vi "Edit Master Gas Mixture.vi"(8 "error in":errorcluster, 11 "Gas Info":T1) -> (0 "error out":errorcluster, 2 "Cancel?":bool, 3 "Gas Info Out":T1)   [LabVIEW 2015]
uses:
  Tests/Controls/Gas Info.ctl
panel:
  in  "Time (s)":u32
  in  "Cancel Button":bool
  in  "OK Button":bool
  in  "PPM":dbl
  in  "Gas":string(combo)
  # "Gas Configuration"
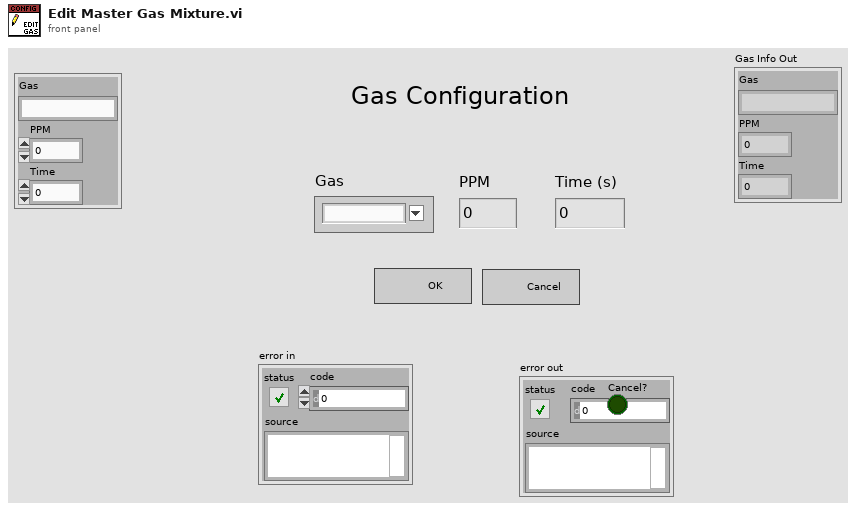
[diagram p1: front panel]
types:
  T1 = typedef "Gas Info.ctl" = cluster{"Gas":string, "PPM":dbl, "Time":u32}
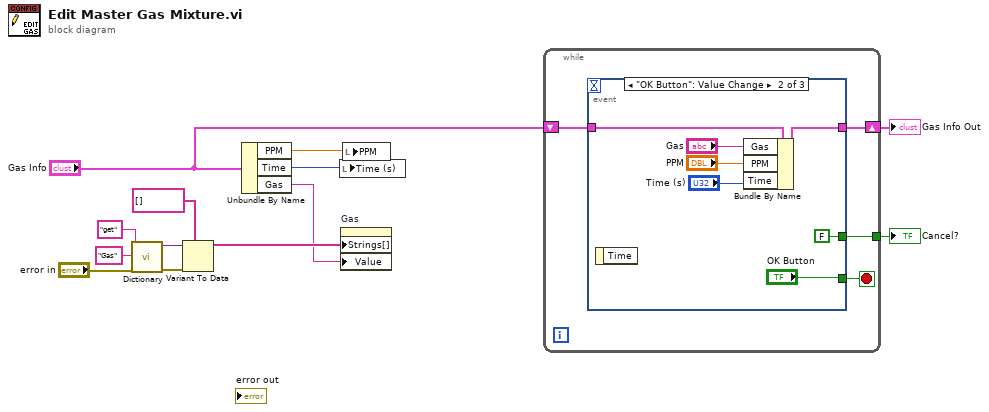
[diagram p0: block diagram]
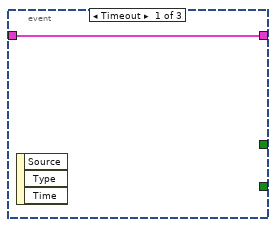
[diagram p2: hidden frame]
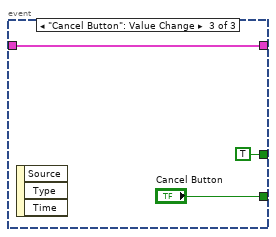
[diagram p3: hidden frame]
diagram:
  n1 = call "Dictionary.vi"("error in"="error in", "Key"="Gas", "Command"="get") -> ("error out"=w11:errorcluster, "Value Out"=w10:variant)  [unwired: 7 in]
  n2 = Variant To Data(error in=w11, type=string[] [] ("Strings []"), Variant=w10) -> (data=w8:string[])  [unwired: 1 out]
  n3 = Unbundle By Name("Gas Info") -> ("PPM"=w5:dbl, "Time"=w3:u32, "Gas"=w6:string)
  n4 = local write "Time (s)"(w3) -> ()
  n5 = property on="Gas" class="CmbBox"("Strings[]"=w8, "Value"=w6) -> ()  [unwired: 2 in, 2 out]
  n6 = local write "PPM"(w5) -> ()
  n7 = while {
    shift-right: [w16] -> w1
    shift-left: "Gas Info" -> [w17]
    tunnel: [w14] -> w4
    stop <- w15 stop-if-true
    n8 = event shown="[1] \"OK Button\": Value Change" {
      selector: _ -> [_ _ _]
      dyn-events: _ -> [_ _ _]
      timeout: _ -> [_ _ _]
      tunnel: w17 -> [w18 w25 w28]
      tunnel: [w18 w24 w28] -> w16
      tunnel: [_ "OK Button" "Cancel Button"] -> w15
      tunnel: [_ FALSE ("OK Button") TRUE ("OK Button")] -> w14
      event Timeout {
        n9 = event-data() -> ()  [unwired: 1 in, 3 out]
      }
      event "OK Button": Value Change {
        n10 = event-data() -> ()  [unwired: 1 in, 1 out]
        n11 = Bundle By Name(cluster=w25, "Gas"="Gas", "PPM"="PPM", "Time"="Time (s)") -> (w24:T1)
      }
      event "Cancel Button": Value Change {
        n12 = event-data() -> ()  [unwired: 1 in, 3 out]
      }
    }
  }
  "Cancel?" <- w4
  "Gas Info Out" <- w1
